vi "ProgressBar init.vi"(8 "error in (no error)":errorcluster, 11 "ProgressBar in":refnum<class "ProgressBar.lvclass">) -> (0 "error out":errorcluster, 3 "ProgressBar out":refnum<class "ProgressBar.lvclass">)   [LabVIEW 2018, in "ProgressBar.lvclass"]
uses:
  ProgressBar.lvclass
  <vilib>/Utility/miscctls.llb/LVPositionTypeDef.ctl
  ProgressBar.lvclass/ProgressBar.ctl
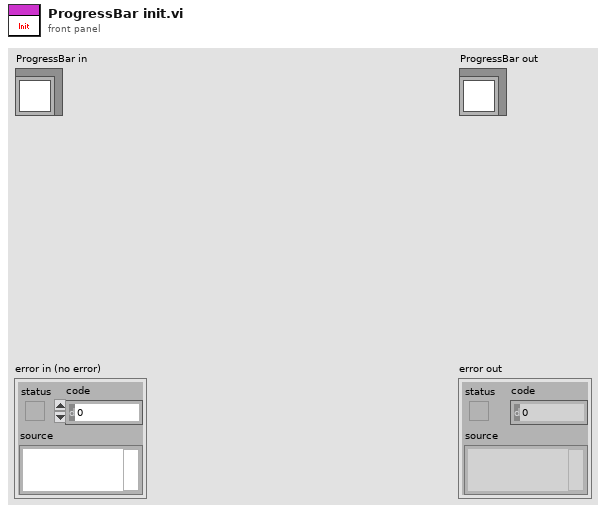
[diagram p1: front panel]
types:
  T1 = typedef "LVPositionTypeDef.ctl" = cluster{"Left":i32, "Top":i32}
  T2 = typedef "LVRectTypeDef.ctl" = cluster{"Left":i16, "Top":i16, "Right":i16, "Bottom":i16}
  T3 = typedef "LVBoundsTypeDef.ctl" = cluster{"Width":u32, "Height":u32}
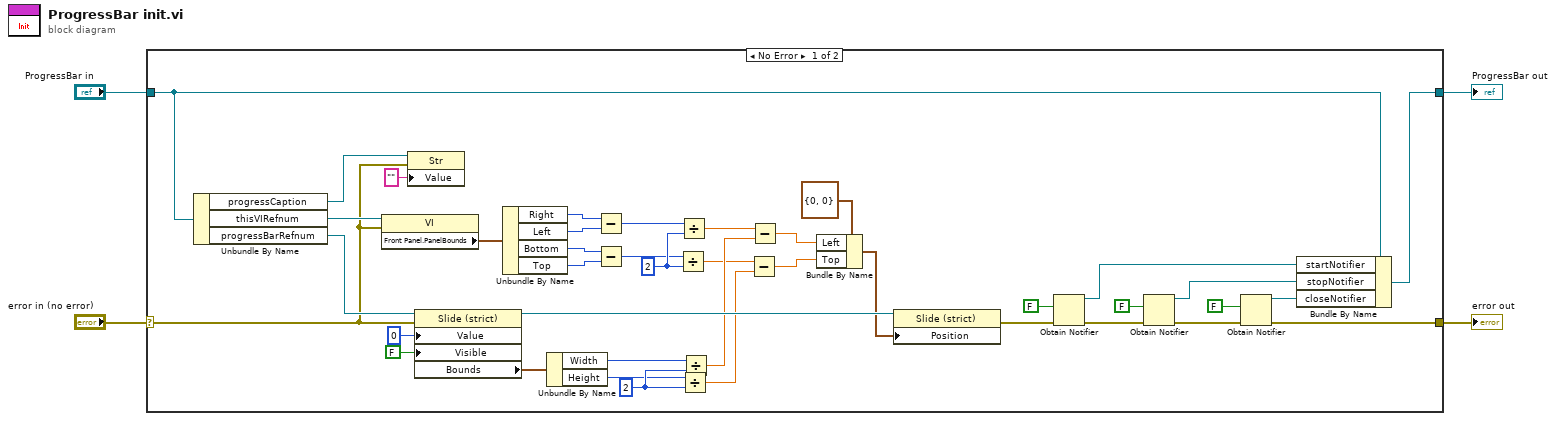
[diagram p0: block diagram]
diagram:
  n1 = case shown="No Error" "error in (no error)" {
    selector: "error in (no error)" -> [w6 w46]
    tunnel: [w36 w46] -> w3
    tunnel: [w35 w45] -> w1
    tunnel: "ProgressBar in" -> [w34 w45]
    frame No Error {
      w19 = u32 2 ("y")
      w23 = u32 2 ("y")
      n2 = Unbundle By Name(w34) -> ("progressCaption"=w7:refnum<vi>, "thisVIRefnum"=w10:refnum<vi>, "progressBarRefnum"=w9:refnum<vi>)
      n3 = property class="VI"(reference=w10, error in=w6) -> ("Front Panel.PanelBounds"=w28:T2)  [unwired: 2 out]
      n4 = property class="Str"(reference=w7, error in=w6, "Value"="") -> ()  [unwired: 2 out]
      n5 = property class="Slide (strict)"(reference=w9, error in=w6, "Value"=0, "Visible"=FALSE) -> (reference out=w31:refnum<vi>, "Bounds"=w20:T3)  [unwired: 1 out]
      n6 = Unbundle By Name(w28) -> ("Right"=w27:i16, "Left"=w26:i16, "Bottom"=w25:i16, "Top"=w24:i16)
      n7 = Unbundle By Name(w20) -> ("Width"=w18:u32, "Height"=w17:u32)
      n8 = Subtract(x=w27, y=w26) -> (x-y=w22:i16)
      n9 = Subtract(x=w25, y=w24) -> (x-y=w21:i16)
      n10 = Divide(x=w21, y=w23) -> (x/y=w14:dbl)
      n11 = Divide(x=w22, y=w23) -> (x/y=w16:dbl)
      n12 = Divide(x=w17, y=w19) -> (x/y=w13:dbl)
      n13 = Divide(x=w18, y=w19) -> (x/y=w15:dbl)
      n14 = Subtract(x=w14, y=w13) -> (x-y=w11:dbl)
      n15 = Subtract(x=w16, y=w15) -> (x-y=w12:dbl)
      n16 = Bundle By Name(cluster=T1 {"Left"=0, "Top"=0} ("Position"), "Left"=w12, "Top"=w11) -> (w29:T1)
      n17 = property class="Slide (strict)"(reference=w31, "Position"=w29) -> (error out=w8:errorcluster)  [unwired: 1 in, 1 out]
      n18 = Obtain Notifier(notification data type=FALSE, error in (no error)=w8) -> (notifier out=w41:refnum<notifier>, error out=w42:errorcluster)  [unwired: 2 in, 1 out]
      n19 = Obtain Notifier(notification data type=FALSE, error in (no error)=w42) -> (notifier out=w38:refnum<notifier>, error out=w39:errorcluster)  [unwired: 2 in, 1 out]
      n20 = Obtain Notifier(notification data type=FALSE, error in (no error)=w39) -> (notifier out=w37:refnum<notifier>, error out=w36:errorcluster)  [unwired: 2 in, 1 out]
      n21 = Bundle By Name(cluster=w34, "startNotifier"=w41, "stopNotifier"=w38, "closeNotifier"=w37) -> (w35:refnum<class "ProgressBar.lvclass">)
    }
    frame Error {
    }
  }
  "error out" <- w3
  "ProgressBar out" <- w1
